vi "Add to Container.vi"(8 "error in (no error)":errorcluster, 10 "Container Enqueuer":refnum<class "Message Enqueuer.lvclass">, 11 "GUI View in":refnum<class "GUI View.lvclass">) -> (0 "error out":errorcluster, 3 "GUI View out":refnum<class "GUI View.lvclass">)   [LabVIEW 2023, in "GUI Views.lvlib" / "GUI View.lvclass"]
uses:
  GUI View.lvclass
  <vilib>/ActorFramework/Message Enqueuer/Message Enqueuer.lvclass
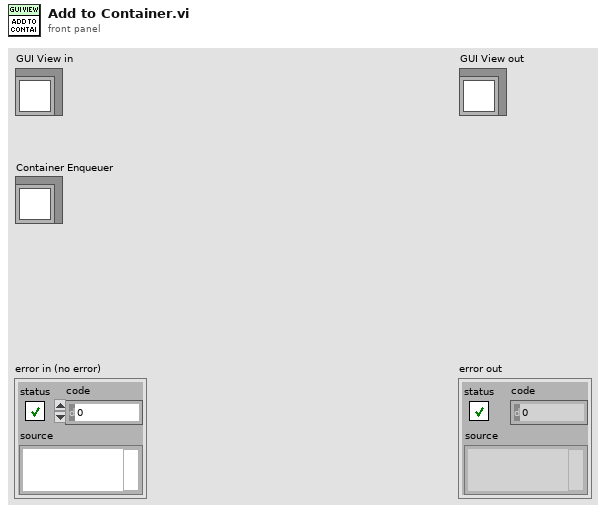
[diagram p1: front panel]
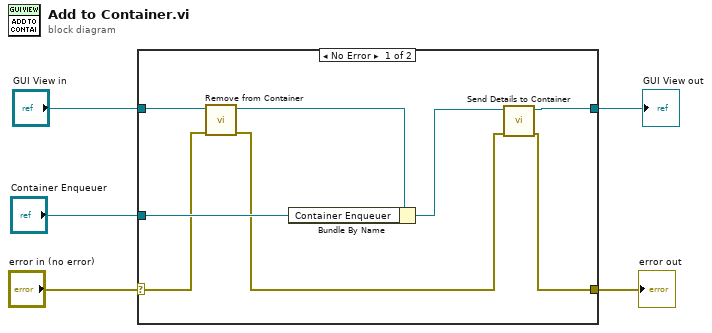
[diagram p0: block diagram]
diagram:
  n1 = case shown="No Error" "error in (no error)" {
    selector: "error in (no error)" -> [w7 w15]
    tunnel: [w10 w15] -> w4
    tunnel: [w11 w14] -> w2
    tunnel: "GUI View in" -> [w9 w14]
    tunnel: "Container Enqueuer" -> [w13 _]
    frame No Error {
      n2 = call "Remove from Container.vi"("error in (no error)"=w7, "GUI View in"=w9) -> ("error out"=w6:errorcluster, "GUI View out"=w8:refnum<class "GUI View.lvclass">)  [unwired: 8 in]
      n3 = Bundle By Name(cluster=w8, "Container Enqueuer"=w13) -> (w12:refnum<class "GUI View.lvclass">)
      n4 = call "Send Details to Container.vi"("error in (no error)"=w6, "GUI View in"=w12) -> ("error out"=w10:errorcluster, "GUI View out"=w11:refnum<class "GUI View.lvclass">)  [unwired: 8 in]
    }
    frame Error {
    }
  }
  "error out" <- w4
  "GUI View out" <- w2
